vi "9239_SampleRates.vi"(9 "error in (no error)":errorcluster, 11 "Data Rate [S/s]":u32) -> (1 "error out":errorcluster, 3 "Data Rate":T1=1 items=["50.000 kS/s (NI 9239)"=1, "25.000 kS/s (NI 9239)"=2, "16.667 kS/s (NI 9239)"=3, "12.500 kS/s (NI 9239)"=4, "10.000 kS/s (NI 9239)"=5, "8.333 kS/s (NI 9239)"=6, "7.143 kS/s (NI 9239)"=7, "6.250 kS/s (NI 9239)"=8, "5.556 kS/s (NI 9239)"=9, "5.000 kS/s (NI 9239)"=10, "4.545 kS/s (NI 9239)"=11, "4.167 kS/s (NI 9239)"=12, "3.846 kS/s (NI 9239)"=13, "3.571 kS/s (NI 9239)"=14, "3.333 kS/s (NI 9239)"=15, "3.125 kS/s (NI 9239)"=16, "2.941 kS/s (NI 9239)"=17, "2.778 kS/s (NI 9239)"=18, "2.632 kS/s (NI 9239)"=19, "2.500 kS/s (NI 9239)"=20, "2.381 kS/s (NI 9239)"=21, "2.273 kS/s (NI 9239)"=22, "2.174 kS/s (NI 9239)"=23, "2.083 kS/s (NI 9239)"=24, "2.000 kS/s (NI 9239)"=25, "1.923 kS/s (NI 9239)"=26, "1.852 kS/s (NI 9239)"=27, "1.786 kS/s (NI 9239)"=28, "1.724 kS/s (NI 9239)"=29, "1.667 kS/s (NI 9239)"=30, "1.613 kS/s (NI 9239)"=31])   [LabVIEW 2017]
uses:
  <vilib>/LabVIEW Targets/FPGA/cRIO/shared/nicrio_ModuleControls/nicrio_cRIO-9239_DataRatesRing.ctl
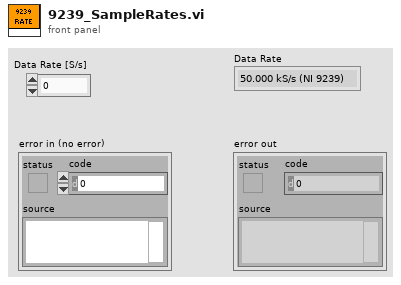
[diagram p1: front panel]
types:
  T1 = typedef "nicrio_cRIO-9239_DataRatesRing.ctl" = u8
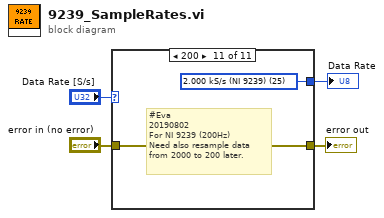
[diagram p0: block diagram]
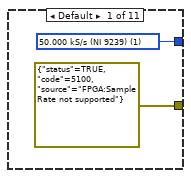
[diagram p2: hidden frame]
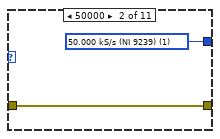
[diagram p3: hidden frame]
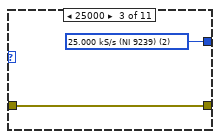
[diagram p4: hidden frame]
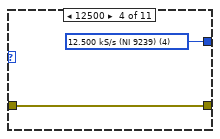
[diagram p5: hidden frame]
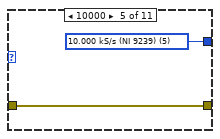
[diagram p6: hidden frame]
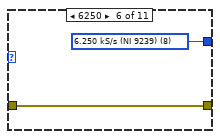
[diagram p7: hidden frame]
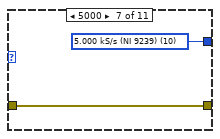
[diagram p8: hidden frame]
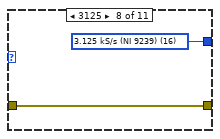
[diagram p9: hidden frame]
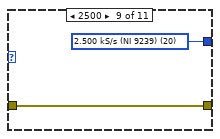
[diagram p10: hidden frame]
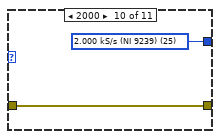
[diagram p11: hidden frame]
diagram:
  n1 = case shown="200" "Data Rate [S/s]" {
    tunnel: "error in (no error)" -> [_ w7 w9 w11 w13 w15 w17 w19 w21 w23 w25]
    tunnel: [errorcluster {"status"=TRUE, "code"=5100, "source"="FPGA:Sample Rate not supported"} ("error IO") w7 w9 w11 w13 w15 w17 w19 w21 w23 w25] -> w2
    tunnel: [w5 w8 w10 w12 w14 w16 w18 w20 w22 w24 w26] -> w1
    frame Default {
      w5 = T1 1 items=["50.000 kS/s (NI 9239)"=1, "25.000 kS/s (NI 9239)"=2, "16.667 kS/s (NI 9239)"=3, "12.500 kS/s (NI 9239)"=4, "10.000 kS/s (NI 9239)"=5, "8.333 kS/s (NI 9239)"=6, "7.143 kS/s (NI 9239)"=7, "6.250 kS/s (NI 9239)"=8, "5.556 kS/s (NI 9239)"=9, "5.000 kS/s (NI 9239)"=10, "4.545 kS/s (NI 9239)"=11, "4.167 kS/s (NI 9239)"=12, "3.846 kS/s (NI 9239)"=13, "3.571 kS/s (NI 9239)"=14, "3.333 kS/s (NI 9239)"=15, "3.125 kS/s (NI 9239)"=16, "2.941 kS/s (NI 9239)"=17, "2.778 kS/s (NI 9239)"=18, "2.632 kS/s (NI 9239)"=19, "2.500 kS/s (NI 9239)"=20, "2.381 kS/s (NI 9239)"=21, "2.273 kS/s (NI 9239)"=22, "2.174 kS/s (NI 9239)"=23, "2.083 kS/s (NI 9239)"=24, "2.000 kS/s (NI 9239)"=25, "1.923 kS/s (NI 9239)"=26, "1.852 kS/s (NI 9239)"=27, "1.786 kS/s (NI 9239)"=28, "1.724 kS/s (NI 9239)"=29, "1.667 kS/s (NI 9239)"=30, "1.613 kS/s (NI 9239)"=31] ("Data Rate")
    }
    frame 50000 {
      w8 = T1 1 items=["50.000 kS/s (NI 9239)"=1, "25.000 kS/s (NI 9239)"=2, "16.667 kS/s (NI 9239)"=3, "12.500 kS/s (NI 9239)"=4, "10.000 kS/s (NI 9239)"=5, "8.333 kS/s (NI 9239)"=6, "7.143 kS/s (NI 9239)"=7, "6.250 kS/s (NI 9239)"=8, "5.556 kS/s (NI 9239)"=9, "5.000 kS/s (NI 9239)"=10, "4.545 kS/s (NI 9239)"=11, "4.167 kS/s (NI 9239)"=12, "3.846 kS/s (NI 9239)"=13, "3.571 kS/s (NI 9239)"=14, "3.333 kS/s (NI 9239)"=15, "3.125 kS/s (NI 9239)"=16, "2.941 kS/s (NI 9239)"=17, "2.778 kS/s (NI 9239)"=18, "2.632 kS/s (NI 9239)"=19, "2.500 kS/s (NI 9239)"=20, "2.381 kS/s (NI 9239)"=21, "2.273 kS/s (NI 9239)"=22, "2.174 kS/s (NI 9239)"=23, "2.083 kS/s (NI 9239)"=24, "2.000 kS/s (NI 9239)"=25, "1.923 kS/s (NI 9239)"=26, "1.852 kS/s (NI 9239)"=27, "1.786 kS/s (NI 9239)"=28, "1.724 kS/s (NI 9239)"=29, "1.667 kS/s (NI 9239)"=30, "1.613 kS/s (NI 9239)"=31] ("Data Rate")
    }
    frame 25000 {
      w10 = T1 2 items=["50.000 kS/s (NI 9239)"=1, "25.000 kS/s (NI 9239)"=2, "16.667 kS/s (NI 9239)"=3, "12.500 kS/s (NI 9239)"=4, "10.000 kS/s (NI 9239)"=5, "8.333 kS/s (NI 9239)"=6, "7.143 kS/s (NI 9239)"=7, "6.250 kS/s (NI 9239)"=8, "5.556 kS/s (NI 9239)"=9, "5.000 kS/s (NI 9239)"=10, "4.545 kS/s (NI 9239)"=11, "4.167 kS/s (NI 9239)"=12, "3.846 kS/s (NI 9239)"=13, "3.571 kS/s (NI 9239)"=14, "3.333 kS/s (NI 9239)"=15, "3.125 kS/s (NI 9239)"=16, "2.941 kS/s (NI 9239)"=17, "2.778 kS/s (NI 9239)"=18, "2.632 kS/s (NI 9239)"=19, "2.500 kS/s (NI 9239)"=20, "2.381 kS/s (NI 9239)"=21, "2.273 kS/s (NI 9239)"=22, "2.174 kS/s (NI 9239)"=23, "2.083 kS/s (NI 9239)"=24, "2.000 kS/s (NI 9239)"=25, "1.923 kS/s (NI 9239)"=26, "1.852 kS/s (NI 9239)"=27, "1.786 kS/s (NI 9239)"=28, "1.724 kS/s (NI 9239)"=29, "1.667 kS/s (NI 9239)"=30, "1.613 kS/s (NI 9239)"=31] ("Data Rate")
    }
    frame 12500 {
      w12 = T1 4 items=["50.000 kS/s (NI 9239)"=1, "25.000 kS/s (NI 9239)"=2, "16.667 kS/s (NI 9239)"=3, "12.500 kS/s (NI 9239)"=4, "10.000 kS/s (NI 9239)"=5, "8.333 kS/s (NI 9239)"=6, "7.143 kS/s (NI 9239)"=7, "6.250 kS/s (NI 9239)"=8, "5.556 kS/s (NI 9239)"=9, "5.000 kS/s (NI 9239)"=10, "4.545 kS/s (NI 9239)"=11, "4.167 kS/s (NI 9239)"=12, "3.846 kS/s (NI 9239)"=13, "3.571 kS/s (NI 9239)"=14, "3.333 kS/s (NI 9239)"=15, "3.125 kS/s (NI 9239)"=16, "2.941 kS/s (NI 9239)"=17, "2.778 kS/s (NI 9239)"=18, "2.632 kS/s (NI 9239)"=19, "2.500 kS/s (NI 9239)"=20, "2.381 kS/s (NI 9239)"=21, "2.273 kS/s (NI 9239)"=22, "2.174 kS/s (NI 9239)"=23, "2.083 kS/s (NI 9239)"=24, "2.000 kS/s (NI 9239)"=25, "1.923 kS/s (NI 9239)"=26, "1.852 kS/s (NI 9239)"=27, "1.786 kS/s (NI 9239)"=28, "1.724 kS/s (NI 9239)"=29, "1.667 kS/s (NI 9239)"=30, "1.613 kS/s (NI 9239)"=31] ("Data Rate")
    }
    frame 10000 {
      w14 = T1 5 items=["50.000 kS/s (NI 9239)"=1, "25.000 kS/s (NI 9239)"=2, "16.667 kS/s (NI 9239)"=3, "12.500 kS/s (NI 9239)"=4, "10.000 kS/s (NI 9239)"=5, "8.333 kS/s (NI 9239)"=6, "7.143 kS/s (NI 9239)"=7, "6.250 kS/s (NI 9239)"=8, "5.556 kS/s (NI 9239)"=9, "5.000 kS/s (NI 9239)"=10, "4.545 kS/s (NI 9239)"=11, "4.167 kS/s (NI 9239)"=12, "3.846 kS/s (NI 9239)"=13, "3.571 kS/s (NI 9239)"=14, "3.333 kS/s (NI 9239)"=15, "3.125 kS/s (NI 9239)"=16, "2.941 kS/s (NI 9239)"=17, "2.778 kS/s (NI 9239)"=18, "2.632 kS/s (NI 9239)"=19, "2.500 kS/s (NI 9239)"=20, "2.381 kS/s (NI 9239)"=21, "2.273 kS/s (NI 9239)"=22, "2.174 kS/s (NI 9239)"=23, "2.083 kS/s (NI 9239)"=24, "2.000 kS/s (NI 9239)"=25, "1.923 kS/s (NI 9239)"=26, "1.852 kS/s (NI 9239)"=27, "1.786 kS/s (NI 9239)"=28, "1.724 kS/s (NI 9239)"=29, "1.667 kS/s (NI 9239)"=30, "1.613 kS/s (NI 9239)"=31] ("Data Rate")
    }
    frame 6250 {
      w16 = T1 8 items=["50.000 kS/s (NI 9239)"=1, "25.000 kS/s (NI 9239)"=2, "16.667 kS/s (NI 9239)"=3, "12.500 kS/s (NI 9239)"=4, "10.000 kS/s (NI 9239)"=5, "8.333 kS/s (NI 9239)"=6, "7.143 kS/s (NI 9239)"=7, "6.250 kS/s (NI 9239)"=8, "5.556 kS/s (NI 9239)"=9, "5.000 kS/s (NI 9239)"=10, "4.545 kS/s (NI 9239)"=11, "4.167 kS/s (NI 9239)"=12, "3.846 kS/s (NI 9239)"=13, "3.571 kS/s (NI 9239)"=14, "3.333 kS/s (NI 9239)"=15, "3.125 kS/s (NI 9239)"=16, "2.941 kS/s (NI 9239)"=17, "2.778 kS/s (NI 9239)"=18, "2.632 kS/s (NI 9239)"=19, "2.500 kS/s (NI 9239)"=20, "2.381 kS/s (NI 9239)"=21, "2.273 kS/s (NI 9239)"=22, "2.174 kS/s (NI 9239)"=23, "2.083 kS/s (NI 9239)"=24, "2.000 kS/s (NI 9239)"=25, "1.923 kS/s (NI 9239)"=26, "1.852 kS/s (NI 9239)"=27, "1.786 kS/s (NI 9239)"=28, "1.724 kS/s (NI 9239)"=29, "1.667 kS/s (NI 9239)"=30, "1.613 kS/s (NI 9239)"=31] ("Data Rate")
    }
    frame 5000 {
      w18 = T1 10 items=["50.000 kS/s (NI 9239)"=1, "25.000 kS/s (NI 9239)"=2, "16.667 kS/s (NI 9239)"=3, "12.500 kS/s (NI 9239)"=4, "10.000 kS/s (NI 9239)"=5, "8.333 kS/s (NI 9239)"=6, "7.143 kS/s (NI 9239)"=7, "6.250 kS/s (NI 9239)"=8, "5.556 kS/s (NI 9239)"=9, "5.000 kS/s (NI 9239)"=10, "4.545 kS/s (NI 9239)"=11, "4.167 kS/s (NI 9239)"=12, "3.846 kS/s (NI 9239)"=13, "3.571 kS/s (NI 9239)"=14, "3.333 kS/s (NI 9239)"=15, "3.125 kS/s (NI 9239)"=16, "2.941 kS/s (NI 9239)"=17, "2.778 kS/s (NI 9239)"=18, "2.632 kS/s (NI 9239)"=19, "2.500 kS/s (NI 9239)"=20, "2.381 kS/s (NI 9239)"=21, "2.273 kS/s (NI 9239)"=22, "2.174 kS/s (NI 9239)"=23, "2.083 kS/s (NI 9239)"=24, "2.000 kS/s (NI 9239)"=25, "1.923 kS/s (NI 9239)"=26, "1.852 kS/s (NI 9239)"=27, "1.786 kS/s (NI 9239)"=28, "1.724 kS/s (NI 9239)"=29, "1.667 kS/s (NI 9239)"=30, "1.613 kS/s (NI 9239)"=31] ("Data Rate")
    }
    frame 3125 {
      w20 = T1 16 items=["50.000 kS/s (NI 9239)"=1, "25.000 kS/s (NI 9239)"=2, "16.667 kS/s (NI 9239)"=3, "12.500 kS/s (NI 9239)"=4, "10.000 kS/s (NI 9239)"=5, "8.333 kS/s (NI 9239)"=6, "7.143 kS/s (NI 9239)"=7, "6.250 kS/s (NI 9239)"=8, "5.556 kS/s (NI 9239)"=9, "5.000 kS/s (NI 9239)"=10, "4.545 kS/s (NI 9239)"=11, "4.167 kS/s (NI 9239)"=12, "3.846 kS/s (NI 9239)"=13, "3.571 kS/s (NI 9239)"=14, "3.333 kS/s (NI 9239)"=15, "3.125 kS/s (NI 9239)"=16, "2.941 kS/s (NI 9239)"=17, "2.778 kS/s (NI 9239)"=18, "2.632 kS/s (NI 9239)"=19, "2.500 kS/s (NI 9239)"=20, "2.381 kS/s (NI 9239)"=21, "2.273 kS/s (NI 9239)"=22, "2.174 kS/s (NI 9239)"=23, "2.083 kS/s (NI 9239)"=24, "2.000 kS/s (NI 9239)"=25, "1.923 kS/s (NI 9239)"=26, "1.852 kS/s (NI 9239)"=27, "1.786 kS/s (NI 9239)"=28, "1.724 kS/s (NI 9239)"=29, "1.667 kS/s (NI 9239)"=30, "1.613 kS/s (NI 9239)"=31] ("Data Rate")
    }
    frame 2500 {
      w22 = T1 20 items=["50.000 kS/s (NI 9239)"=1, "25.000 kS/s (NI 9239)"=2, "16.667 kS/s (NI 9239)"=3, "12.500 kS/s (NI 9239)"=4, "10.000 kS/s (NI 9239)"=5, "8.333 kS/s (NI 9239)"=6, "7.143 kS/s (NI 9239)"=7, "6.250 kS/s (NI 9239)"=8, "5.556 kS/s (NI 9239)"=9, "5.000 kS/s (NI 9239)"=10, "4.545 kS/s (NI 9239)"=11, "4.167 kS/s (NI 9239)"=12, "3.846 kS/s (NI 9239)"=13, "3.571 kS/s (NI 9239)"=14, "3.333 kS/s (NI 9239)"=15, "3.125 kS/s (NI 9239)"=16, "2.941 kS/s (NI 9239)"=17, "2.778 kS/s (NI 9239)"=18, "2.632 kS/s (NI 9239)"=19, "2.500 kS/s (NI 9239)"=20, "2.381 kS/s (NI 9239)"=21, "2.273 kS/s (NI 9239)"=22, "2.174 kS/s (NI 9239)"=23, "2.083 kS/s (NI 9239)"=24, "2.000 kS/s (NI 9239)"=25, "1.923 kS/s (NI 9239)"=26, "1.852 kS/s (NI 9239)"=27, "1.786 kS/s (NI 9239)"=28, "1.724 kS/s (NI 9239)"=29, "1.667 kS/s (NI 9239)"=30, "1.613 kS/s (NI 9239)"=31] ("Data Rate")
    }
    frame 2000 {
      w24 = T1 25 items=["50.000 kS/s (NI 9239)"=1, "25.000 kS/s (NI 9239)"=2, "16.667 kS/s (NI 9239)"=3, "12.500 kS/s (NI 9239)"=4, "10.000 kS/s (NI 9239)"=5, "8.333 kS/s (NI 9239)"=6, "7.143 kS/s (NI 9239)"=7, "6.250 kS/s (NI 9239)"=8, "5.556 kS/s (NI 9239)"=9, "5.000 kS/s (NI 9239)"=10, "4.545 kS/s (NI 9239)"=11, "4.167 kS/s (NI 9239)"=12, "3.846 kS/s (NI 9239)"=13, "3.571 kS/s (NI 9239)"=14, "3.333 kS/s (NI 9239)"=15, "3.125 kS/s (NI 9239)"=16, "2.941 kS/s (NI 9239)"=17, "2.778 kS/s (NI 9239)"=18, "2.632 kS/s (NI 9239)"=19, "2.500 kS/s (NI 9239)"=20, "2.381 kS/s (NI 9239)"=21, "2.273 kS/s (NI 9239)"=22, "2.174 kS/s (NI 9239)"=23, "2.083 kS/s (NI 9239)"=24, "2.000 kS/s (NI 9239)"=25, "1.923 kS/s (NI 9239)"=26, "1.852 kS/s (NI 9239)"=27, "1.786 kS/s (NI 9239)"=28, "1.724 kS/s (NI 9239)"=29, "1.667 kS/s (NI 9239)"=30, "1.613 kS/s (NI 9239)"=31] ("Data Rate")
    }
    frame 200 {
      w26 = T1 25 items=["50.000 kS/s (NI 9239)"=1, "25.000 kS/s (NI 9239)"=2, "16.667 kS/s (NI 9239)"=3, "12.500 kS/s (NI 9239)"=4, "10.000 kS/s (NI 9239)"=5, "8.333 kS/s (NI 9239)"=6, "7.143 kS/s (NI 9239)"=7, "6.250 kS/s (NI 9239)"=8, "5.556 kS/s (NI 9239)"=9, "5.000 kS/s (NI 9239)"=10, "4.545 kS/s (NI 9239)"=11, "4.167 kS/s (NI 9239)"=12, "3.846 kS/s (NI 9239)"=13, "3.571 kS/s (NI 9239)"=14, "3.333 kS/s (NI 9239)"=15, "3.125 kS/s (NI 9239)"=16, "2.941 kS/s (NI 9239)"=17, "2.778 kS/s (NI 9239)"=18, "2.632 kS/s (NI 9239)"=19, "2.500 kS/s (NI 9239)"=20, "2.381 kS/s (NI 9239)"=21, "2.273 kS/s (NI 9239)"=22, "2.174 kS/s (NI 9239)"=23, "2.083 kS/s (NI 9239)"=24, "2.000 kS/s (NI 9239)"=25, "1.923 kS/s (NI 9239)"=26, "1.852 kS/s (NI 9239)"=27, "1.786 kS/s (NI 9239)"=28, "1.724 kS/s (NI 9239)"=29, "1.667 kS/s (NI 9239)"=30, "1.613 kS/s (NI 9239)"=31] ("Data Rate")
      # "#Eva\n20190802\nFor NI 9239 (200Hz)\nNeed also resample data \nfrom 2000 to 200 later."
    }
  }
  "error out" <- w2
  "Data Rate" <- w1
